vi "DecipherWhoWins.vi"(11 "A":string) -> (3 "Enum":enum16{"NOT Defined", "I LOSE", "DRAW", "I WIN"}(ring))   [LabVIEW 2021, in "2022.lvlib"]
uses:
  2022.lvlib
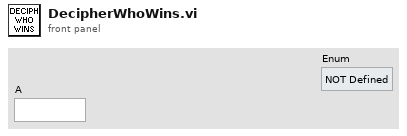
[diagram p1: front panel]
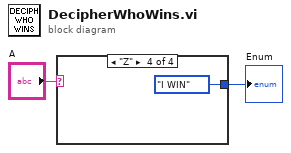
[diagram p0: block diagram]
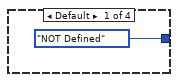
[diagram p2: hidden frame]
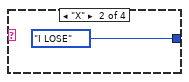
[diagram p3: hidden frame]
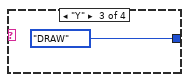
[diagram p4: hidden frame]
diagram:
  n1 = case shown="\"Z\"" "A" {
    tunnel: [enum16{"NOT Defined", "I LOSE", "DRAW", "I WIN"}."NOT Defined" enum16{"NOT Defined", "I LOSE", "DRAW", "I WIN"}."I LOSE" enum16{"NOT Defined", "I LOSE", "DRAW", "I WIN"}."DRAW" enum16{"NOT Defined", "I LOSE", "DRAW", "I WIN"}."I WIN"] -> w1
    frame Default {
    }
    frame "X" {
    }
    frame "Y" {
    }
    frame "Z" {
    }
  }
  "Enum" <- w1
